vi "HovaCAL point purge.vi"(6 "Sprachliste":string[][](array[string]), 8 "error in (no error)":errorcluster caption="Fehler (Eingang, kein Fehler)", 9 "letzter Punkt":bool, 10 "Punkt":i32, 11 "Timer (Eingang)":timestamp) -> (0 "error out":errorcluster caption="Fehler (Ausgang)", 1 "Status":string, 2 "Aktion out":T1, 3 "Timer (Ausgang)":timestamp, 4 "Sprachliste out":string[][](array[string]))   [LabVIEW 2020, in "EPA 1065.lvlib" / "HovaCAL Interference verificaton.lvlib"]
uses:
  HovaCAL Interference verificaton.lvlib
  Aktion Test.ctl
  Linearisierung V2/SpanEinstellungen/Aktion FGV GD Errors sammeln.ctl
  Linearisierung V2/SpanEinstellungen/GD Info Cluster.ctl
  Linearisierung V2/LIN ErrorCluster.ctl
  Linearisierung V2/SpanEinstellungen/SpanEinstellungen.lvlib
  Linearisierung V2/Linearisierung v2.lvlib
  Linearisierung V2/Gasteiler/HovaCAL_Interface/HovaCAL_Interface.lvlib
  Linearisierung V2/Gasteiler/Gasteiler.lvlib
  Sprachverwaltung/Sprachverwaltung.lvlib
  Linearisierung V2/Gasteiler/HovaCal/Aktion_FGV_Betriebsdaten.ctl
  Linearisierung V2/Gasteiler/HovaCal/HovaCal.lvlib
  Linearisierung V2/Gasteiler/HovaCal/Aktion_FGV_Kom.ctl
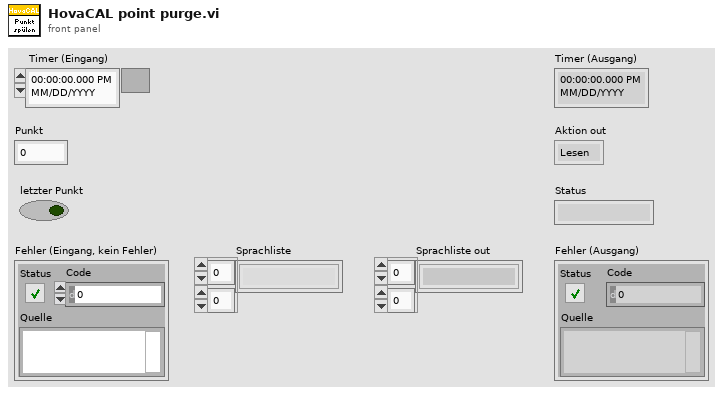
[diagram p1: front panel]
types:
  T1 = typedef "EPA 1065.lvlib/HovaCAL Interference verificaton.lvlib/Aktion Test.ctl" = enum16{"Lesen", "ini", "ini-Warten-Stabil", "Warten-Stabil", "ini-warten-aufzeichnen", "Warten-Aufzeichnen", "aufzeichnen", "fertig", "spülen", "abbrechen"}
  T2 = typedef "Linearisierung v2.lvlib/SpanEinstellungen.lvlib/GD Info Cluster.ctl" = cluster{"Wobei":string, "Status":string, "Errors":T3, "Empfangsdaten":string[], "Zeitstempel":string}
  T3 = typedef "Linearisierung v2.lvlib/LIN ErrorCluster.ctl" = cluster{"Störung Kommunikation":bool, "Pressure carrier gas":bool, "Pressure diluted gas":bool, "Outlet Pressure":bool, "SNOX before SAIR":bool, "Störung Gasteiler":bool}
  T4 = typedef "Linearisierung v2.lvlib/SpanEinstellungen.lvlib/Aktion FGV GD Errors sammeln.ctl" = enum16{"lesen", "init", "GD Infos sammeln", "Kalibrierinfos sammeln", "Test Data", "GD Infos selektiv sammeln"}
  T5 = typedef "Linearisierung v2.lvlib/Gasteiler.lvlib/HovaCal.lvlib/Aktion_FGV_Kom.ctl" = enum16{"Initialisieren", "Betriebsparameter", "Gase", "Vaporizer", "Dynamische Werte", "Beenden", "Com ändern", "Gase init"}
  T6 = typedef "Linearisierung v2.lvlib/Gasteiler.lvlib/HovaCal.lvlib/Aktion_FGV_Betriebsdaten.ctl" = enum16{"Lesen", "Sollwerte schreiben", "Sollwerte lesen", "Gase schreiben", "Gase lesen", "Dynamische Werte", "GaseRef", "Gase aendern"}
  T7 = typedef "Linearisierung v2.lvlib/Gasteiler.lvlib/HovaCal.lvlib/Betriebsdaten.ctl" = cluster{"Gesamtdurchfluss":dbl, "Eingangskonzentration \nTrägergas":dbl, "Eingangskonzentration\nKomponente 1":dbl, "Eingangskonzentration \nKomponente 2":dbl, "Ausgangskonzentration \nKomponente 1 ":dbl, "Ausgangskonzentration\nKomponente 2":dbl, "l/min -> ml/min":bool, "N2 %->ppm":bool, "Komp1 ppm->%":bool, "Komp2ppm->%":bool, "Sollkomp1ppm->%":bool, "Sollkomp2ppm->%":bool}
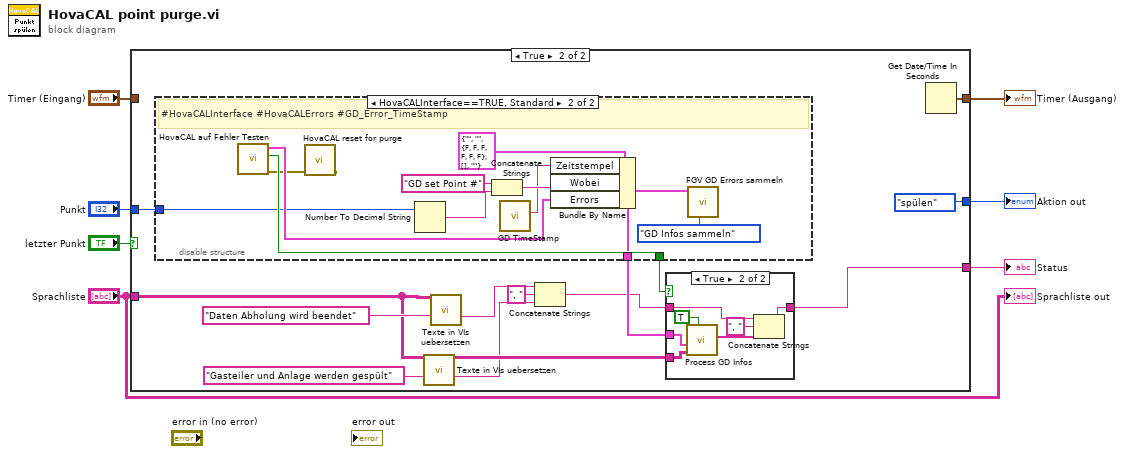
[diagram p0: block diagram]
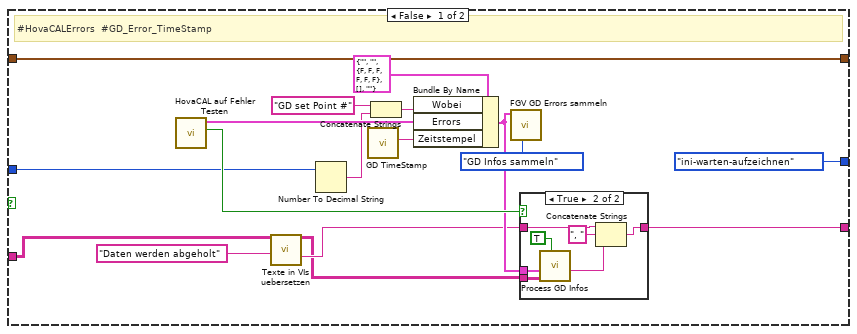
[diagram p2: hidden frame]
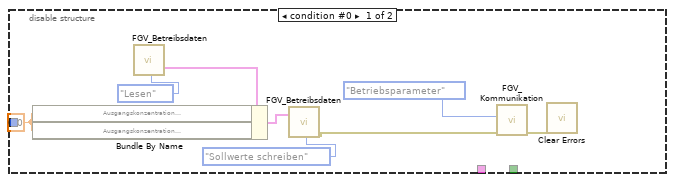
[diagram p5: hidden frame]
diagram:
  n1 = case shown="True" "letzter Punkt" {
    tunnel: [Aktion_Test."ini-warten-aufzeichnen" ("Enum") Aktion_Test."spülen" ("Enum")] -> w1
    tunnel: [w19 w41] -> w6
    tunnel: "Timer (Eingang)" -> [w24 _]
    tunnel: [w24 w46] -> w7
    tunnel: "Sprachliste" -> [w10 w43]
    tunnel: "Punkt" -> [w14 w38]
    frame False {
      # "#HovaCALErrors  #GD_Error_TimeStamp"
      n2 = call "HovaCAL auf Fehler Testen.vi"() -> ("Error"=w20:bool, "LNI Error Ausgangs-Cluster"=w18:T3)  [unwired: 9 in, 1 out]
      n3 = call "Texte in VIs uebersetzen.vi"("Sprachliste"=w10, "String zum Übersetzen"="Daten werden abgeholt") -> ("Sprachliste out"=w9:string[][], "String zum Übersetzen"=w11:string)  [unwired: 9 in, 3 out]
      n4 = Number To Decimal String(number=w14) -> (decimal integer string=w15:string)  [unwired: 1 in]
      n5 = call "GD TimeStamp.vi"() -> ("date/time string"=w13:string)  [unwired: 10 in, 1 out]
      n6 = Concatenate Strings("GD set Point #" ("Status"), w15) -> (w16:string)
      n7 = Bundle By Name(cluster=T2 {"Wobei"="", "Status"="", "Errors"={"Störung Kommunikation"=FALSE, "Pressure carrier gas"=FALSE, "Pressure diluted gas"=FALSE, "Outlet Pressure"=FALSE, "SNOX before SAIR"=FALSE, "Störung Gasteiler"=FALSE}, "Empfangsdaten"=[], "Zeitstempel"=""} ("GD Info-Cluster in"), "Wobei"=w16, "Errors"=w18, "Zeitstempel"=w13) -> (w17:T2)
      n8 = call "FGV GD Errors sammeln.vi"("Aktion"=Aktion_FGV_GD_Errors_sammeln."GD Infos sammeln", "GD Info-Cluster in"=w17) -> ()  [unwired: 7 in, 3 out]
      n9 = case shown="True" w20 {
        tunnel: [w25 w27] -> w19
        tunnel: w9 -> [_ w32]
        tunnel: w17 -> [_ w31]
        tunnel: w11 -> [w25 w28]
        frame False {
        }
        frame True {
          n10 = call "Process GD Infos.vi"("show Status even if no Error"=TRUE, "Sprachliste"=w32, "GD Info-Cluster in"=w31) -> ("GD Infos"=w26:string)  [unwired: 6 in, 2 out]
          n11 = Concatenate Strings(w28, ", " ("String"), w26) -> (w27:string)
        }
      }
    }
    frame True {
      n12 = disable-structure shown="HovaCALInterface==TRUE, Standard" {
        disable-tunnel: [_ w70] -> w42
        disable-tunnel: [_ w68] -> w39
        disable-tunnel: w38 -> [_ w66]
        frame condition #0 {
          w61 = 0.0 ("Eingangskonzentration \nKomponente 2")
          n13 = call "FGV_Betreibsdaten.vi"("Enum"=Aktion_FGV_Betriebsdaten."Lesen") -> ("Sollwert für Vergleich"=w60:T7)  [unwired: 11 in, 7 out]
          n14 = Bundle By Name(cluster=w60, "Ausgangskonzentration \nKomponente 1"=w61, "Ausgangskonzentration\nKomponente 2"=w61) -> (w62:T7)
          n15 = call "FGV_Betreibsdaten.vi"("Sollwert schreiben"=w62, "Enum"=Aktion_FGV_Betriebsdaten."Sollwerte schreiben") -> ("error out"=w55:errorcluster)  [unwired: 10 in, 7 out]
          n16 = call "FGV_Kommunikation.vi"("error in"=w55, "Aktion"=Aktion_FGV_Kom."Betriebsparameter" ("Enum")) -> ("error out"=w56:errorcluster)  [unwired: 5 in, 4 out]
          n17 = call <vilib>:"Clear Errors.vi"("error in (no error)"=w56) -> ()  [unwired: 5 in, 2 out]
        }
        frame condition #1 (active) {
          # "#HovaCALInterface #HovaCALErrors #GD_Error_TimeStamp"
          n18 = call "HovaCAL auf Fehler Testen.vi"() -> ("error out"=w63:errorcluster, "Error"=w70:bool, "LNI Error Ausgangs-Cluster"=w69:T3)  [unwired: 9 in]
          n19 = call "HovaCAL reset for purge.vi"("Fehler (Eingang, kein Fehler)"=w63) -> ()  [unwired: 10 in, 1 out]
          n20 = Number To Decimal String(number=w66) -> (decimal integer string=w65:string)  [unwired: 1 in]
          n21 = Concatenate Strings("GD set Point #" ("Status"), w65) -> (w67:string)
          n22 = call "GD TimeStamp.vi"() -> ("date/time string"=w64:string)  [unwired: 10 in, 1 out]
          n23 = Bundle By Name(cluster=T2 {"Wobei"="", "Status"="", "Errors"={"Störung Kommunikation"=FALSE, "Pressure carrier gas"=FALSE, "Pressure diluted gas"=FALSE, "Outlet Pressure"=FALSE, "SNOX before SAIR"=FALSE, "Störung Gasteiler"=FALSE}, "Empfangsdaten"=[], "Zeitstempel"=""} ("GD Info-Cluster in"), "Zeitstempel"=w64, "Wobei"=w67, "Errors"=w69) -> (w68:T2)
          n24 = call "FGV GD Errors sammeln.vi"("Aktion"=Aktion_FGV_GD_Errors_sammeln."GD Infos sammeln", "GD Info-Cluster in"=w68) -> ()  [unwired: 7 in, 3 out]
        }
      }
      n25 = call "Texte in VIs uebersetzen.vi"("Sprachliste"=w43, "String zum Übersetzen"="Gasteiler und Anlage werden gespült" ("String 2 hinzufügen")) -> ("Sprachliste out"=w40:string[][], "String zum Übersetzen"=w37:string)  [unwired: 9 in, 3 out]
      n26 = call "Texte in VIs uebersetzen.vi"("Sprachliste"=w43, "String zum Übersetzen"="Daten Abholung wird beendet" ("String 1 hinzufügen")) -> ("String zum Übersetzen"=w35:string)  [unwired: 9 in, 4 out]
      n27 = Concatenate Strings(w35, ", " ("String"), w37) -> (w36:string)
      n28 = case shown="True" w42 {
        tunnel: w36 -> [w47 w49]
        tunnel: [w47 w50] -> w41
        tunnel: w40 -> [_ w53]
        tunnel: w39 -> [_ w54]
        frame False {
        }
        frame True {
          n29 = call "Process GD Infos.vi"("show Status even if no Error"=TRUE, "Sprachliste"=w53, "GD Info-Cluster in"=w54) -> ("Array (Ausgang)"=w48:string[])  [unwired: 6 in, 2 out]
          n30 = Concatenate Strings(w49, ", " ("String"), w48) -> (w50:string)
        }
      }
      n31 = Get Date/Time In Seconds() -> (seconds since 1Jan1904=w46:timestamp)
    }
  }
  "Timer (Ausgang)" <- w7
  "Status" <- w6
  "Aktion out" <- w1
  "Sprachliste out" <- "Sprachliste"
